vi "test_TxUDP-RxUDP - Multiple Boards - Float_64.vi"(8 "error in":errorcluster, 11 "reference in":refnum<class "AIM ARINC 664 Loopback.lvclass">) -> (0 "error out":errorcluster, 3 "reference out":refnum<class "AIM ARINC 664 Loopback.lvclass">)   [LabVIEW 2020, in "AIM ARINC 664 Loopback.lvclass"]
uses:
  AIM ARINC 664 Loopback.lvclass
  C:/Program Files/National Instruments/LabVIEW 2024/vi.lib/NI/VeriStand Custom Device Testing Tools/VeriStandTestCase/VeriStandTestCase.lvclass
  AIM ARINC 664 Loopback.lvclass/AIM ARINC 664 Loopback.ctl
  b47c41b5-a02e-49d5-b852-4e28f097d7ad.vi
  6a3dd3ed-914d-4d14-bf18-724521aa5e28.vi
  8abe1e9f-12f7-4d29-bb0e-ea5e1950c3f4.vi
  NationalInstruments.VeriStand.SystemDefinitionAPI
  <vilib>/addons/_JKI Toolkits/VI Tester/TestCase.llb/TestCase.lvclass
  Scripting/AIM ARINC 664 Scripting.lvlib
  Import/AIM ARINC 664 Import.lvlib
  <vilib>/NI/VeriStand Custom Device Testing Tools/VeriStandTestCase/VeriStandTestCase.lvclass
  C:/Program Files/National Instruments/LabVIEW 2024/vi.lib/addons/_JKI Toolkits/VI Tester/TestCase.llb/TestCase.lvclass
panel:
  out "resulting string":string
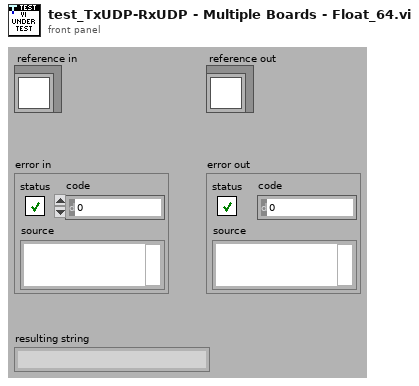
[diagram p1: front panel]
types:
  T1 = typedef "Custom Device API.lvlib/Custom Device Item Ref.ctl" = u64
  T2 = typedef "AIM ARINC 664 Import.lvlib/Board Top Level Configuration.ctl" = cluster{"boardSetup":T3, "portConfiguration":T4[]}
  T3 = typedef "AIM ARINC 664 Import.lvlib/board_setup.ctl" = cluster{"boardId":u32, "portSpeed":u32, "portConfig":u32}
  T4 = typedef "AIM ARINC 664 Import.lvlib/port_configuration.ctl" = cluster{"portSetup":T5, "Tx_Generic":T6[], "Rx_Monitor":cluster{"DefaultCronoMode":u32, "GlbMonBufferSizeIn":u32, "CaptureMode":u32, "MaxFileSizeMB":u32, "Strobe":u32, "TriggerPosition":u32}[], "Tx_UDP":cluster{"tx_udp_setup":cluster{"VlId":i32, "Bag":i32, "NetSelect":u32, "domainID":u8, "sideID":u8, "locationID":u8, "interfaceID":u8, "NumOfSubVl":u16, "Skew":u32, "MaxFrameLength":u32, "FrameBufferSize":u32}, "commPorts":T14[], "sapPorts":T15[]}[], "Rx_UDP":cluster{"Tx_UDP":T16, "commPorts":T17[], "sapPorts":T18[]}[]}
  T5 = typedef "AIM ARINC 664 Import.lvlib/port_setup.ctl" = cluster{"port Id":u32, "redundant":bool}
  T6 = typedef "AIM ARINC 664 Import.lvlib/session_tx_generic.ctl" = cluster{"tx_generic_setup":T7, "Frame Headers":T8[]}
  T7 = typedef "AIM ARINC 664 Import.lvlib/tx_generic_setup.ctl" = cluster{"QueueSizeIn":u32, "Count":i32, "StartMode":i32}
  T8 = typedef "AIM ARINC 664 Import.lvlib/frame_tx_generic.ctl" = cluster{"FrameID":string, "PayloadID":string, "Frame header":cluster{"FrameStartMode":i32, "InterFrameGap":i32, "PacketGroupWaitTime":i32, "NetSelect":u32, "PayloadBufferMode":i32, "PayloadGenerationMode":i32, "PhysErrorInjection":i32, "PreambleCount":i32, "SequenceNumberInit":T9, "SequenceNumberOffset":T10, "Skew":i32}, "Parameters":T11[]}
  T9 = typedef "AIM ARINC 664 Import.lvlib/frame_tx_generic_seqNumberInit.ctl" = i32
  T10 = typedef "AIM ARINC 664 Import.lvlib/frame_tx_generic_seqNumberOffset.ctl" = i32
  T11 = typedef "AIM ARINC 664 Import.lvlib/frame_parameter.ctl" = cluster{"name":string, "default value":dbl, "unit":string, "Parameter":T12}
  T12 = typedef "AIM ARINC 664 Import.lvlib/frame_parameter_definition.ctl" = cluster{"start index":i32, "size":i32, "encoding":T13, "signed":bool, "scale multiplier":dbl, "scale offset":dbl}
  T13 = typedef "Encoding (Arinc664).ctl" = u16
  T14 = typedef "AIM ARINC 664 Import.lvlib/port_tx_udp_comm.ctl" = cluster{"PayloadID":string, "partitionID":u8, "UdpSrcPort":u16, "UdpDstPort":u16, "PortType":enum16{"FDX_UDP_SAMPLING", "FDX_UDP_QUEUING"}, "SubVIId":u32, "UdpNumBufMessages":u32, "UdpMaxMessageSize":u32, "UdpSamplingRate":u32, "Parameters":T11[]}
  T15 = typedef "AIM ARINC 664 Import.lvlib/port_tx_udp_sap.ctl" = cluster{"PayloadID":string, "SubVlId":u8, "UdpSrcPort":u16, "UdpNumBufMessages":u32, "UdpMaxMessageSize":u32, "partitionID":u8, "domainID":u8, "sideID":u8, "locationID":u8, "interfaceID":u8, "Parameters":T11[]}
  T16 = typedef "AIM ARINC 664 Import.lvlib/rx_udp_setup.ctl" = cluster{"VerificationMode":u32, "Bag":u32, "Jitter":u32, "MaxFrameLength":u32, "MaxSkew":u32, "VLBufSize":u32, "FilterMode":u32, "FilterPosition":u32, "Padding":u32, "FilterMask":u32, "FilterData":u32, "MinFrameLength":u32, "VlId":u16, "VLRange":u32}
  T17 = typedef "AIM ARINC 664 Import.lvlib/port_rx_udp_comm.ctl" = cluster{"PayloadID":string, "domainID":u8, "sideID":u8, "locationID":u8, "partitionID":u8, "UdpSrcPort":u16, "UdpDstPort":u16, "PortType":enum16{"FDX_UDP_SAMPLING", "FDX_UDP_QUEUING"}, "SubVIId":u32, "UdpNumBufMessages":u32, "UdpMaxMessageSize":u32, "UdpSamplingRate":u32, "Parameters":T11[]}
  T18 = typedef "AIM ARINC 664 Import.lvlib/port_rx_udp_sap.ctl" = cluster{"PayloadID":string, "UdpDstPort":u16, "UdpNumBufMessages":u32, "UdpMaxMessageSize":u32, "Parameters":T11[]}
  T19 = typedef "Payload Map.ctl" = map{string, T20}
  T20 = typedef "Payload Record Type.ctl" = cluster{"Data":u8[], "Type of Frame":T21}
  T21 = typedef "Type of Payload.ctl" = u16
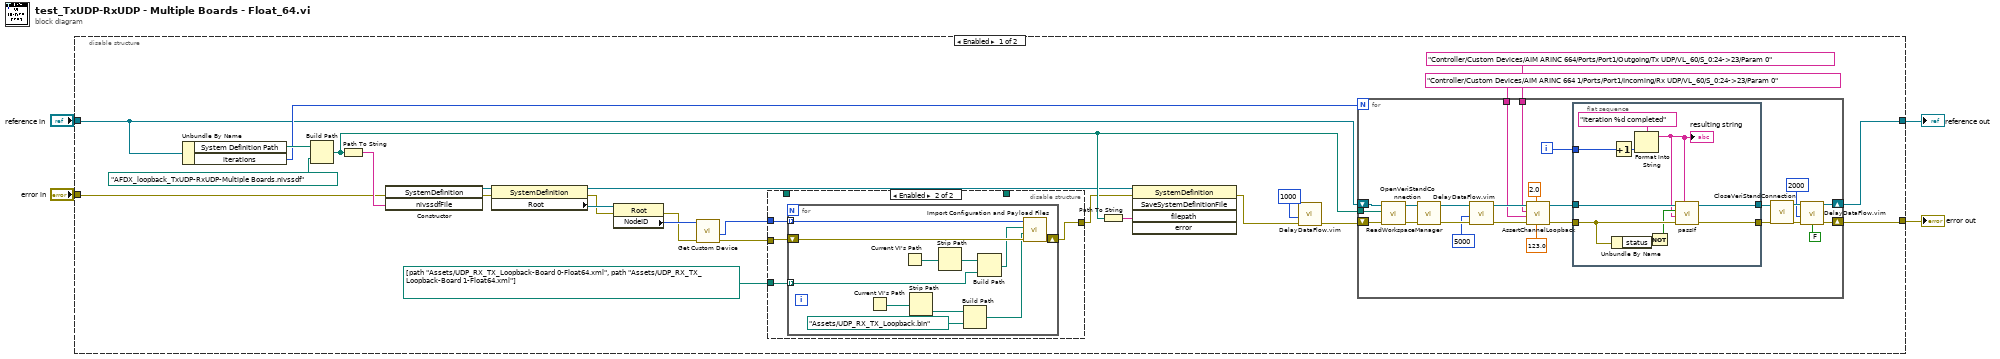
[diagram p0: block diagram]
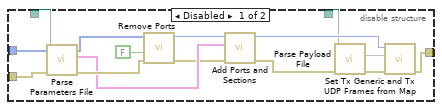
[diagram p2: hidden frame]
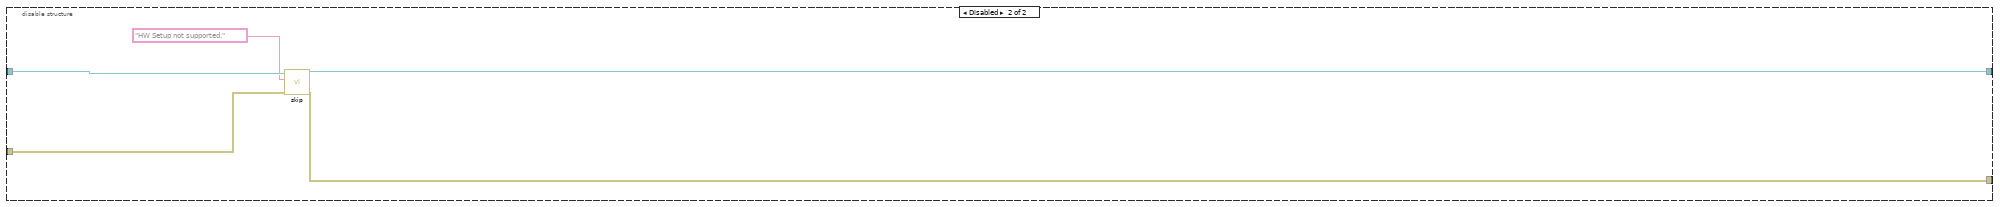
[diagram p3: hidden frame]
diagram:
  n1 = disable-structure shown="Enabled" {
    disable-tunnel: "reference in" -> [w8 w97]
    disable-tunnel: "error in" -> [w7 w96]
    disable-tunnel: [w28 w95] -> w2
    disable-tunnel: [w27 w94] -> w1
    frame Enabled {
      n2 = Unbundle By Name(w8) -> ("System Definition Path"=w30:path, "iterations"=w14:i32)
      n3 = Build Path(base path=w30, name or relative path=path "AFDX_loopback_TxUDP-RxUDP-Multiple Boards.nivssdf") -> (appended path=w25:path)
      n4 = Path To String(path=w25) -> (string=w26:string)
      n5 = constructor class="SystemDefinition"(error in=w7, "nivssdfFile"=w26) -> (reference out=w24:refnum<k24>, error out=w22:errorcluster)  [unwired: 2 in, 2 out]
      n6 = property class="SystemDefinition"(reference=w24, error in=w22) -> (reference out=w19:refnum<k24>, error out=w21:errorcluster, "Root"=w23:refnum<k24>)
      n7 = property class="Root"(reference=w23, error in=w21) -> (error out=w16:errorcluster, "NodeID"=w17:u64)  [unwired: 1 out]
      n8 = call "Get Custom Device.vi"("error in"=w16, "custom device ref in"=w17) -> ("error out"=w15:errorcluster, "Item Refs"=w6:T1[])  [unwired: 5 in, 3 out]
      n9 = disable-structure shown="Enabled" {
        disable-tunnel: w6 -> [w76 w80]
        disable-tunnel: w15 -> [w68 w81]
        disable-tunnel: _ -> [w66 _]
        disable-tunnel: _ -> [w65 _]
        disable-tunnel: [w64 w79] -> w20
        disable-tunnel: path[] [path "Assets/UDP_RX_TX_Loopback-Board 0-Float64.xml", path "Assets/UDP_RX_TX_Loopback-Board 1-Float64.xml"] -> [_ w78]
        frame Disabled {
          n10 = call "Parse Parameters File.vi"("error in"=w68, "path to XML document"=w65) -> ("error out"=w77:errorcluster, "board configuration out"=w74:T2)  [unwired: 7 in, 1 out]
          n11 = call "Remove Ports.vi"("error in"=w77, "refresh?"=FALSE, "Custom device Ref"=w76) -> ("error out"=w73:errorcluster, "Custom device Ref out"=w75:T1)  [unwired: 7 in]
          n12 = call "Add Ports and Sections.vi"("error in"=w73, "board configuration in"=w74, "custom device ref"=w75) -> ("error out"=w72:errorcluster, "custom device ref out"=w67:T1)  [unwired: 7 in]
          n13 = call "Parse Payload File.vi"("error in"=w72, "frame array path in"=w66) -> ("error out"=w71:errorcluster, "Map"=w70:T19)  [unwired: 7 in, 1 out]
          n14 = call "Set Tx Generic and Tx UDP Frames from Map.vi"("error in"=w71, "payload map"=w70, "custom device ref"=w67) -> ("error out"=w64:errorcluster)  [unwired: 7 in, 1 out]
        }
        frame Enabled {
          n15 = for {
            shift-right: [w91] -> w79
            shift-left: w81 -> [w92]
            tunnel: w78 -> [w84] mode=indexing
            tunnel: w80 -> [w83] mode=indexing
            n16 = Current VI's Path() -> (path=w89:path)
            n17 = Current VI's Path() -> (path=w86:path)
            n18 = Strip Path(path=w89) -> (stripped path=w90:path)  [unwired: 1 out]
            n19 = Strip Path(path=w86) -> (stripped path=w87:path)  [unwired: 1 out]
            n20 = Build Path(base path=w90, name or relative path=path "Assets/UDP_RX_TX_Loopback.bin") -> (appended path=w88:path)
            n21 = Build Path(base path=w87, name or relative path=w84) -> (appended path=w85:path)
            n22 = call "Import Configuration and Payload Files.vi"("error in"=w92, "payload file path"=w88, "parameters configuration file path"=w85, "custom device ref"=w83) -> ("error out"=w91:errorcluster)  [unwired: 6 in, 1 out]
          }
        }
      }
      n23 = Path To String(path=w25) -> (string=w18:string)
      n24 = invoke class="SystemDefinition" method="SaveSystemDefinitionFile"(reference=w19, error in=w20, "filepath"=w18) -> (error out=w13:errorcluster)  [unwired: 2 in, 4 out]
      n25 = call "DelayDataFlow.vim"("value in"=w13, "milliseconds to wait"=u32 1000) -> ("value out"=w12:errorcluster)  [unwired: 2 in, 1 out]
      n26 = for {
        N: w14 -> [_]
        tunnel: w25 -> [w46]
        shift-right: [w51] -> w27
        shift-left: w8 -> [w53]
        shift-right: [w40] -> w28
        shift-left: w12 -> [w47]
        tunnel: "Controller/Custom Devices/AIM ARINC 664 1/Ports/Port1/Incoming/Rx UDP/VL_60/S_0:24->23/Param 0" -> [w32]
        tunnel: "Controller/Custom Devices/AIM ARINC 664/Ports/Port1/Outgoing/Tx UDP/VL_60/S_0:24->23/Param 0" -> [w31]
        i -> [w34]
        n27 = call-dynamic "OpenVeriStandConnection.vi"("error in (no error)"=w47, "System Definition File"=w46, "VeriStand Test Case in"=w53) -> ("error out"=w52:errorcluster, "VeriStand Test Case out"=w50:refnum<class "AIM ARINC 664 Loopback.lvclass">)  [unwired: 6 in, 1 out]
        n28 = call-dynamic "ReadWorkspaceManager.vi"("error in (no error)"=w52, "VeriStand Test Case in"=w50) -> ("error out"=w49:errorcluster, "VeriStand Test Case out"=w44:refnum<class "AIM ARINC 664 Loopback.lvclass">)  [unwired: 7 in, 1 out]
        n29 = call "DelayDataFlow.vim"("value in"=w49, "milliseconds to wait"=u32 5000) -> ("value out"=w45:errorcluster)  [unwired: 2 in, 1 out]
        n30 = call <vilib>:"AssertChannelLoopback.vi"("Value"=123.0, "Timeout (1 second)"=2.0, "error in (no error)"=w45, "Read Channel"=w32, "Write Channel"=w31, "VeriStand Test Case in"=w44) -> ("error out"=w35:errorcluster, "VeriStand Test Case out"=w33:refnum<class "AIM ARINC 664 Loopback.lvclass">)  [unwired: 4 in]
        n31 = flat-sequence {
          tunnel: [w63] -> w37
          tunnel: [w62] -> w36
          tunnel: w35 -> [w61]
          tunnel: w34 -> [w57]
          tunnel: w33 -> [w55]
          frame #0 {
            n32 = Unbundle By Name(w61) -> ("status"=w60:bool)
            n33 = Increment(x=w57) -> (x+1=w56:i32)
            n34 = Format Into String(format string="Iteration %d completed", w56) -> (resulting string=w54:string)  [unwired: 2 in, 1 out]
            "resulting string" <- w54
            n35 = Not(x=w60) -> (.not. x?=w59:bool)
            n36 = call-dynamic "passIf.vi"("custom report message (\"\")"=w54, "error in (no error)"=w61, "message (\"\")"=w54, "pass"=w59, "TestCase in"=w55) -> ("error out"=w62:errorcluster, "TestCase out"=w63:refnum<class "AIM ARINC 664 Loopback.lvclass">)  [unwired: 5 in]
          }
        }
        n37 = call-dynamic "CloseVeriStandConnection.vi"("error in (no error)"=w36, "VeriStand Test Case in"=w37) -> ("error out"=w41:errorcluster, "VeriStand Test Case out"=w51:refnum<class "AIM ARINC 664 Loopback.lvclass">)  [unwired: 8 in]
        n38 = call "DelayDataFlow.vim"("value in"=w41, "milliseconds to wait"=u32 2000, "no delay on error (T)"=FALSE) -> ("value out"=w40:errorcluster)  [unwired: 1 in, 1 out]
      }
    }
    frame Disabled {
      n39 = call <vilib>:"skip.vi"("error in (no error)"=w96, "skipMessage"="HW Setup not supported.", "TestCase in"=w97) -> ("error out"=w95:errorcluster, "TestCase out"=w94:refnum<class "AIM ARINC 664 Loopback.lvclass">)  [unwired: 7 in]
    }
  }
  "error out" <- w2
  "reference out" <- w1
